vi "Optimize Path Limits.vi"(8 "max dist":dbl, 9 "accuracy":dbl=0.1, 10 "path params":T2={"Sample Period (s)"=0.0, "Limits"={"Velocity (fps)"=5.0, "Acceleration (fps^2)"=0.0, "Jerk (fps^3)"=0.0}, "Conditions"={"vInitial (fps)"=0.0, "vFinal (fps)"=0.0}, "Angluar Accelerations"={"Angular \nAccelerations"=[], "Override Limits?"=[]}}, 11 "path pts":cluster{"x":dbl, "y":dbl, "th":dbl}[](array[cluster])) -> (2 "fastest time (s)":dbl, 3 "path output":T1)   [LabVIEW 2019]
uses:
  types/path_params.ctl
panel:
  out "Array":u32[](array[numeric])
  out "sum":u32
  out "x-y 2":u32
  out "x-y":u32
  out "Numeric":i32
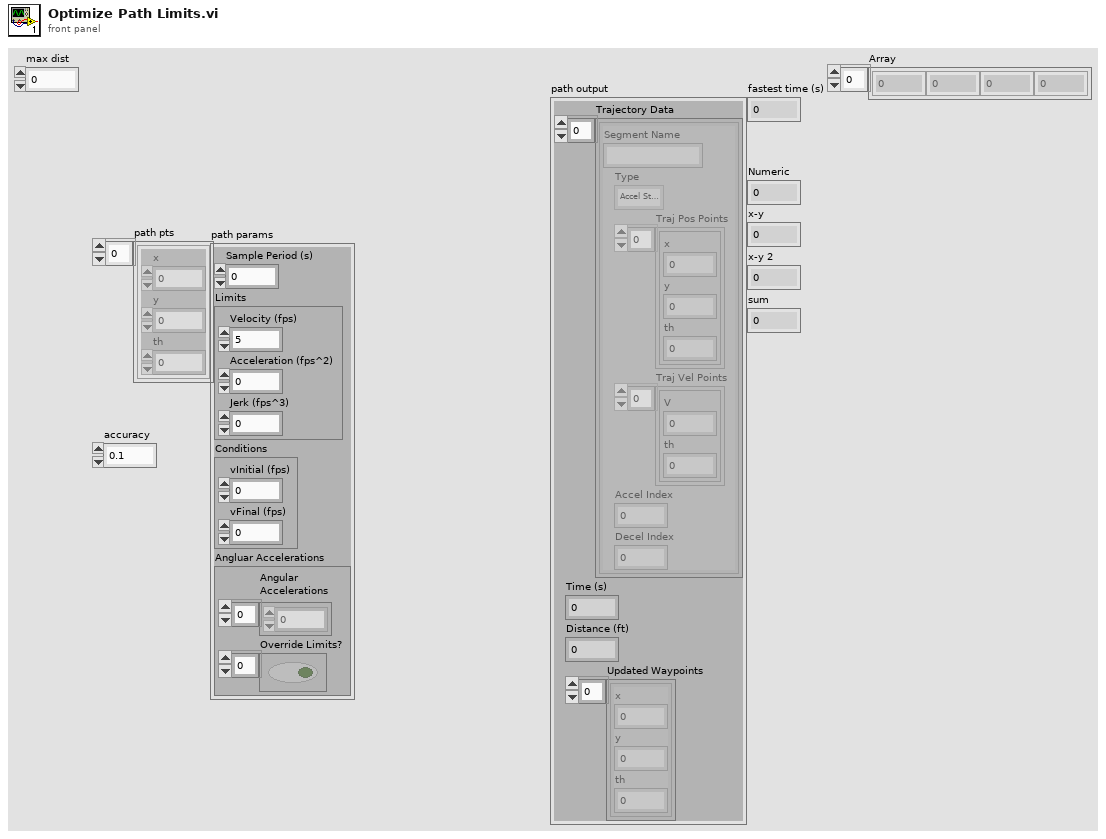
[diagram p1: front panel]
types:
  T1 = cluster{"Trajectory Data":cluster{"Segment Name":string, "Type":enum16{"Accel Straight", "Const Straight", "Blend", "Circle"}, "Traj Pos Points":cluster{"x":dbl, "y":dbl, "th":dbl}[], "Traj Vel Points":cluster{"V":dbl, "th":dbl}[], "Accel Index":i32, "Decel Index":i32}[], "Time (s)":dbl, "Distance (ft)":dbl, "Updated Waypoints":cluster{"x":dbl, "y":dbl, "th":dbl}[]}
  T2 = typedef "path_params.ctl" = cluster{"Sample Period (s)":dbl, "Limits":cluster{"Velocity (fps)":dbl, "Acceleration (fps^2)":dbl, "Jerk (fps^3)":dbl}, "Conditions":cluster{"vInitial (fps)":dbl, "vFinal (fps)":dbl}, "Angluar Accelerations":cluster{"Angular \nAccelerations":dbl[], "Override Limits?":bool[]}}
  T3 = cluster{"Velocity (fps)":dbl, "Acceleration (fps^2)":dbl, "Jerk (fps^3)":dbl}
  T4 = cluster{"vInitial (fps)":dbl, "vFinal (fps)":dbl}
  T5 = cluster{"Angular \nAccelerations":dbl[], "Override Limits?":bool[]}
  T6 = cluster{dbl, "Acceleration (fps^2)":dbl, "Jerk (fps^3)":dbl}
  T7 = cluster{"Segment Name":string, "Type":enum16{"Accel Straight", "Const Straight", "Blend", "Circle"}, "Traj Pos Points":cluster{"x":dbl, "y":dbl, "th":dbl}[], "Traj Vel Points":cluster{"V":dbl, "th":dbl}[], "Accel Index":i32, "Decel Index":i32}[]
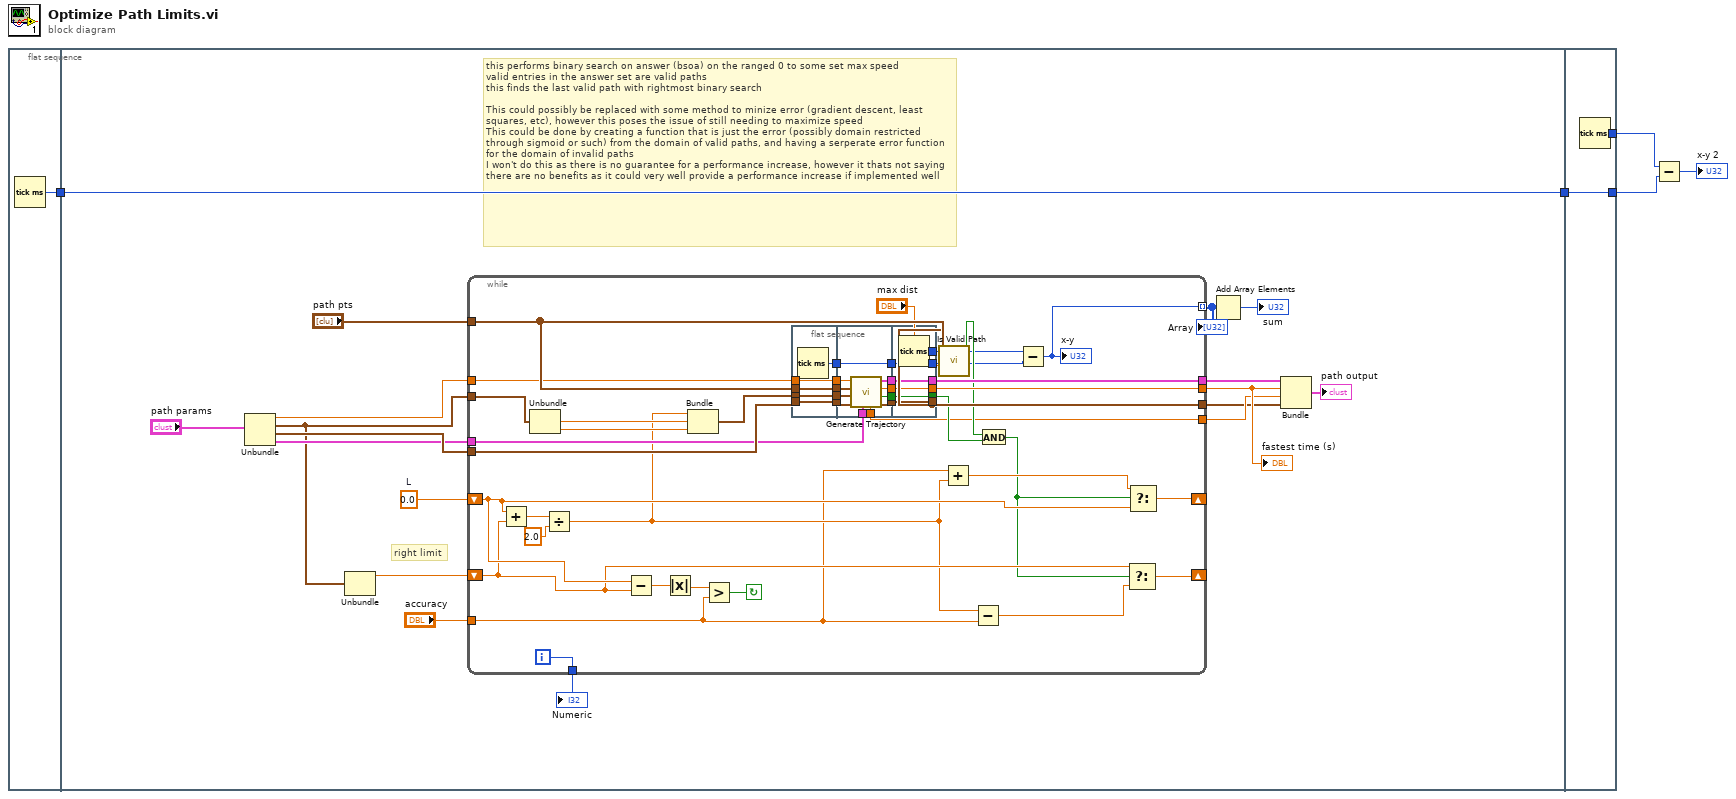
[diagram p0: block diagram]
diagram:
  n1 = flat-sequence {
    tunnel: [w6] -> w2
    tunnel: [w9] -> w3
    tunnel: w2 -> [w9]
    tunnel: [w91] -> w5
    tunnel: [w90] -> w4
    tunnel: w3 -> [w90]
    frame #0 {
      n2 = Tick Count (ms)() -> (millisecond timer value=w6:u32)
    }
    frame #1 {
      w19 = 0.0  # L
      # "right limit"
      # "this performs binary search on answer (bsoa) on the ranged 0 to some set max speed\nvalid entries in the answer set are valid paths\nthis finds the last valid path with rightmost binary search\n\nThis could possibly be replaced with some method to minize error (gradient descent, least squares, etc), however this poses the issue of still needing to maximize speed\nThis could be done by creating a function that is just the error (possibly domain restricted through sigmoid or such) from the domain of valid paths, and having a serperate error function for the domain of invalid paths\nI won't do this as there is no guarantee for a performance increase, however it thats not saying there are no benefits as it could very well provide a performance increase if implemented well"
      n3 = Unbundle("path params") -> ("Sample Period (s)"=w22:dbl, "Limits"=w17:T3, "Conditions"=w21:T4, "Angluar Accelerations"=w20:T5)
      n4 = Unbundle(w17) -> ("Velocity (fps)"=w16:dbl)  [unwired: 2 out]
      n5 = while {
        tunnel: "path pts" -> [w67]
        tunnel: w22 -> [w66]
        tunnel: w21 -> [w65]
        tunnel: w20 -> [w64]
        tunnel: "accuracy" -> [w45]
        shift-right: [w58] -> _
        shift-left: w19 -> [w57]
        shift-right: [w56] -> _
        shift-left: w16 -> [w55]
        tunnel: w17 -> [w53]
        tunnel: [w49] -> w12
        tunnel: [w48] -> w14
        tunnel: [w47] -> w15
        tunnel: [w40] -> w13
        tunnel: [w39] -> w10
        tunnel: [w25] -> w8 mode=indexing
        i -> [w39]
        stop <- w59 continue-if-true
        n6 = Add(x=w57, y=w55) -> (x+y=w63:dbl)
        n7 = Unbundle(w53) -> ("Acceleration (fps^2)"=w52:dbl, "Jerk (fps^3)"=w51:dbl)  [unwired: 1 out]
        n8 = Divide(x=w63, y=2.0) -> (x/y=w46:dbl)
        n9 = Subtract(x=w57, y=w55) -> (x-y=w61:dbl)
        n10 = Absolute Value(x=w61) -> (abs(x)=w60:dbl)
        n11 = Bundle(w46, "Acceleration (fps^2)"=w52, "Jerk (fps^3)"=w51) -> (w50:T6)  [unwired: 1 in]
        n12 = Greater?(x=w60, y=w45) -> (0:w59:bool)
        n13 = flat-sequence {
          tunnel: w50 -> [w69]
          tunnel: w65 -> [w70]
          tunnel: w66 -> [w71]
          tunnel: w67 -> [w72]
          tunnel: [w72] -> w33
          tunnel: [w71] -> w32
          tunnel: [w70] -> w31
          tunnel: [w69] -> w30
          tunnel: [w68] -> w26
          tunnel: w64 -> [w80]
          tunnel: [w74] -> w40
          tunnel: [w78] -> w37
          tunnel: [w77] -> w36
          tunnel: [w76] -> w35
          tunnel: [w75] -> w34
          tunnel: w33 -> [w83]
          tunnel: w32 -> [w82]
          tunnel: w31 -> [w81]
          tunnel: w30 -> [w79]
          tunnel: [w73] -> w27
          tunnel: w26 -> [w73]
          tunnel: [w86] -> w42
          tunnel: [w87] -> w47
          tunnel: [w88] -> w48
          tunnel: [w89] -> w49
          tunnel: w37 -> [w89]
          tunnel: w36 -> [w88]
          tunnel: w35 -> [w87]
          tunnel: w34 -> [w86]
          tunnel: [w85] -> w29
          tunnel: [w84] -> w28
          tunnel: w27 -> [w84]
          frame #0 {
            n14 = Tick Count (ms)() -> (millisecond timer value=w68:u32)
          }
          frame #1 {
            n15 = call "Generate Trajectory.vi"("Angular Accelerations"=w80, "Conditions"=w81, "Limits"=w79, "WayPoints"=w83, "Sample Period (s)"=w82) -> ("Updated Waypoints"=w78:cluster{"x":dbl, "y":dbl, "th":dbl}[], "Valid"=w75:bool, "Time (s)"=w77:dbl, "Trajectory Data"=w76:T7, "Distance (ft)"=w74:dbl)  [unwired: 2 in]
          }
          frame #2 {
            n16 = Tick Count (ms)() -> (millisecond timer value=w85:u32)
          }
        }
        n17 = call "Is Valid Path.vi"("max dist"="max dist", "Waypoints"=w49, "ball pts"=w67) -> ("is valid?"=w43:bool)  [unwired: 8 in]
        n18 = Add(x=w45, y=w46) -> (x+y=w44:dbl)
        n19 = Subtract(x=w46, y=w45) -> (x-y=w54:dbl)
        n20 = And(x=w43, y=w42) -> (x .and. y?=w41:bool)
        n21 = Subtract(x=w29, y=w28) -> (x-y=w25:u32)
        "x-y" <- w25
        n22 = Select(t=w55, s=w41, f=w54) -> (s? t:f=w56:dbl)
        n23 = Select(t=w44, s=w41, f=w57) -> (s? t:f=w58:dbl)
      }
      "fastest time (s)" <- w14
      "Numeric" <- w10
      "Array" <- w8
      n24 = Add Array Elements(numeric array=w8) -> (sum=→"sum":u32)
      n25 = Bundle("Trajectory Data"=w15, "Time (s)"=w14, "Distance (ft)"=w13, "Updated Waypoints"=w12) -> (→"path output":T1)  [unwired: 1 in]
    }
    frame #2 {
      n26 = Tick Count (ms)() -> (millisecond timer value=w91:u32)
    }
  }
  n27 = Subtract(x=w5, y=w4) -> (x-y=→"x-y 2":u32)
